vi "Hadamard.vi"(4 "Wire in":T1) -> (1 "Wire out":T1)   [LabVIEW 2016]
uses:
  TypeDefs/Circuit Cluster.ctl
  Classes/GateAbst/GateAbst.lvclass
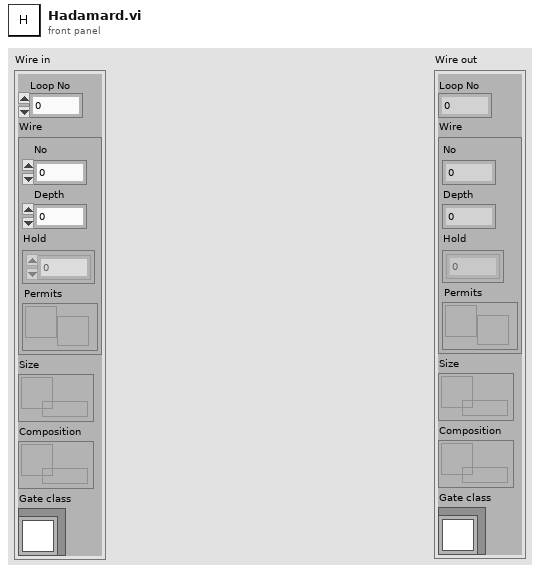
[diagram p1: front panel]
types:
  T1 = typedef "Circuit Cluster.ctl" = cluster{"Loop No":i32, "Wire":cluster{"No":i32, "Depth":i32, "Hold":i32[][], "Permits":refnum<notifier>}, "Size":refnum<queue>, "Composition":refnum<queue>, "Gate class":refnum<class "GateAbst.lvclass">}
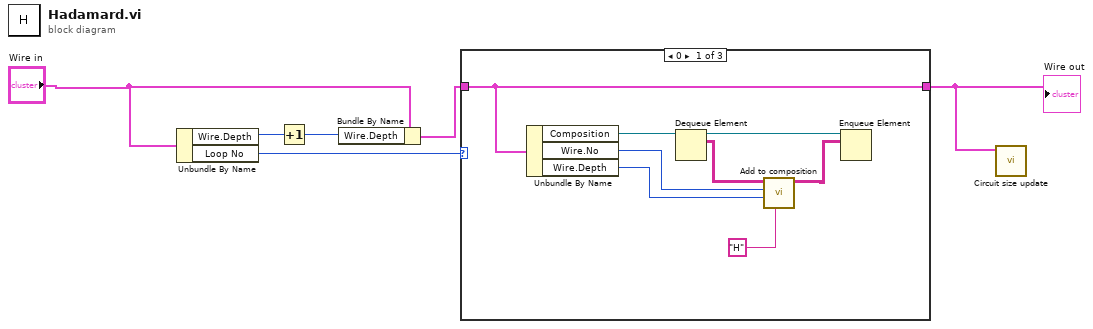
[diagram p0: block diagram]
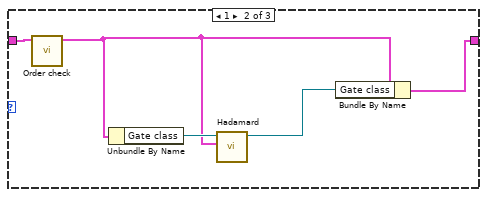
[diagram p2: hidden frame]
diagram:
  n1 = Unbundle By Name("Wire in") -> ("Wire.Depth"=w6:i32, "Loop No"=w1:i32)
  n2 = Increment(x=w6) -> (x+1=w5:i32)
  n3 = Bundle By Name(cluster="Wire in", "Wire.Depth"=w5) -> (w4:T1)
  n4 = case shown="0" w1 {
    tunnel: [w7 w15 w20] -> w2
    tunnel: w4 -> [w7 w16 w20]
    frame 0 {
      n5 = Unbundle By Name(w7) -> ("Composition"=w13:refnum<queue>, "Wire.No"=w12:i32, "Wire.Depth"=w11:i32)
      n6 = Dequeue Element(queue=w13) -> (queue out=w14:refnum<queue>, element=w10:string[][])  [unwired: 2 in, 2 out]
      n7 = call "Add to composition.vi"("Gate name"="H", "Wire depth"=w11, "Wire No"=w12, "Composition in"=w10) -> ("Composition out"=w8:string[][])  [unwired: 7 in]
      n8 = Enqueue Element(queue=w14, element=w8) -> ()  [unwired: 2 in, 3 out]
    }
    frame 1 {
      n9 = call "Order check.vi"("Wire in in"=w16) -> ("Wire out"=w17:T1)  [unwired: 10 in]
      n10 = Unbundle By Name(w17) -> ("Gate class"=w19:refnum<class "GateAbst.lvclass">)
      n11 = call-dynamic "Hadamard.vi"("Wire in"=w17, "GateAbst in"=w19) -> ("GateAbst out"=w18:refnum<class "GateAbst.lvclass">)  [unwired: 8 in, 1 out]
      n12 = Bundle By Name(cluster=w17, "Gate class"=w18) -> (w15:T1)
    }
    frame Default {
    }
  }
  "Wire out" <- w2
  n13 = call "Circuit size update.vi"("Wire in"=w2) -> ()  [unwired: 11 in]
